vi "PointerArray_Clear.vi"(3 "Pointer Array":refnum<class "_Pointer.lvclass">[](array[class])) -> (1 "Pointer Array Out":refnum<class "_Pointer.lvclass">[](array[class]))   [LabVIEW 2020, in "WavBuf.lvclass"]
uses:
  WavBuf/WavBuf.lvclass
  Pointer/_Pointer.lvclass
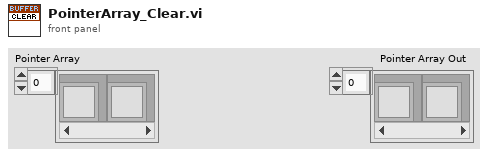
[diagram p1: front panel]
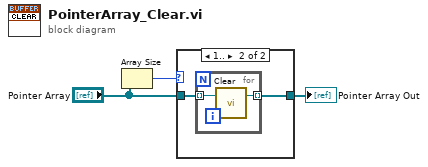
[diagram p0: block diagram]
diagram:
  n1 = Array Size(array="Pointer Array") -> (size(s)=w3:i32)
  n2 = case shown="1.." w3 {
    tunnel: "Pointer Array" -> [w4 w6]
    tunnel: [w4 w5] -> w1
    frame ..0 {
    }
    frame 1.. {
      n3 = for {
        tunnel: w6 -> [w8] mode=indexing
        tunnel: [w7] -> w5 mode=indexing
        n4 = call-dynamic "Clear.vi"("((Pointer)) in"=w8) -> ("((Pointer)) out"=w7:refnum<class "_Pointer.lvclass">)  [unwired: 2 in]
      }
    }
  }
  "Pointer Array Out" <- w1
